vi "DeltaE(1976).vi"(1 "L*a*b* Colors":T1) -> (0 "DeltaE":dbl)   [LabVIEW 2013]
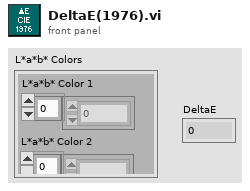
[diagram p1: front panel]
types:
  T1 = cluster{"L*a*b* Color 1":dbl[], "L*a*b* Color 2":dbl[]}
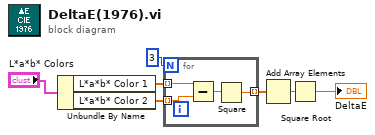
[diagram p0: block diagram]
diagram:
  n1 = Unbundle By Name("L*a*b* Colors") -> ("L*a*b* Color 1"=w5:dbl[], "L*a*b* Color 2"=w4:dbl[])
  n2 = for {
    N: 3 -> [_]
    tunnel: w5 -> [w10] mode=indexing
    tunnel: w4 -> [w11] mode=indexing
    tunnel: [w8] -> w3 mode=indexing
    n3 = Subtract(x=w10, y=w11) -> (x-y=w9:dbl)
    n4 = Square(x=w9) -> (x^2=w8:dbl)
  }
  n5 = Add Array Elements(numeric array=w3) -> (sum=w2:dbl)
  n6 = Square Root(x=w2) -> (sqrt(x)=→"DeltaE":dbl)
